vi "CAPCartTopLevelV2.vi"() -> ()   [LabVIEW 2020]
uses:
  <vilib>/Utility/file.llb/Read Delimited Spreadsheet (string).vi
  BK Precision 4050B Series/BK Precision 4050B Series.lvlib
  consol_upload3 2020/consol_upload3 2020/Program Files/National Instruments/LabVIEW 2021/instr.lib/BK Precision 9200 Series/BK Precision 9200 Series.lvlib
  CAPCart LabVIEW/Marlin/Marlin.lvlib
  Ocean Optics 2000 4000/Ocean Optics 2000 4000.lvlib
panel:
  in  "Flow Controller":refnum<visa-resource-name>="Alicat"
  in  "Enable Strobe (Disabled)":bool
  out "Spectral Waveform":cluster{dbl[], dbl[]}(graph)
  in  "Stop":bool
  in  "Spectrometer":refnum<visa-resource-name>
  out "Frequency Command":string
  out "Voltage Command":string
  out "XYZ Command":string
  out "Flow Command":string
  in  "Time per measurement (ms)":u32
  in  "?":bool
  in  "File path (dialog if empty)":path
  in  "3D Printer":refnum<visa-resource-name>
  in  "Voltage Limit (66V)":dbl=66.0 format="%.2f"
  in  "Enable OVP (T: Enable) 2":bool=TRUE
  in  "Current Limit (1.0 A)":dbl=1.0 format="%.3g"
  in  "Power Supply":refnum<visa-resource-name>
  in  "Function Generator 2":refnum<visa-resource-name>="COM9"
  in  "Amplitude  2":dbl=1.0 format="%#.3f"
  in  "DC Offset (0.00 V)":dbl
  in  "Pulse Width/Duty (20%)":dbl=20.0 format="%.3g"
  # "Plasma and Electric Space Propulsion Lab\nOregon State University\nAlexander Reed & Blake Haist\n\nCAPCartTopLevelRev5.14"
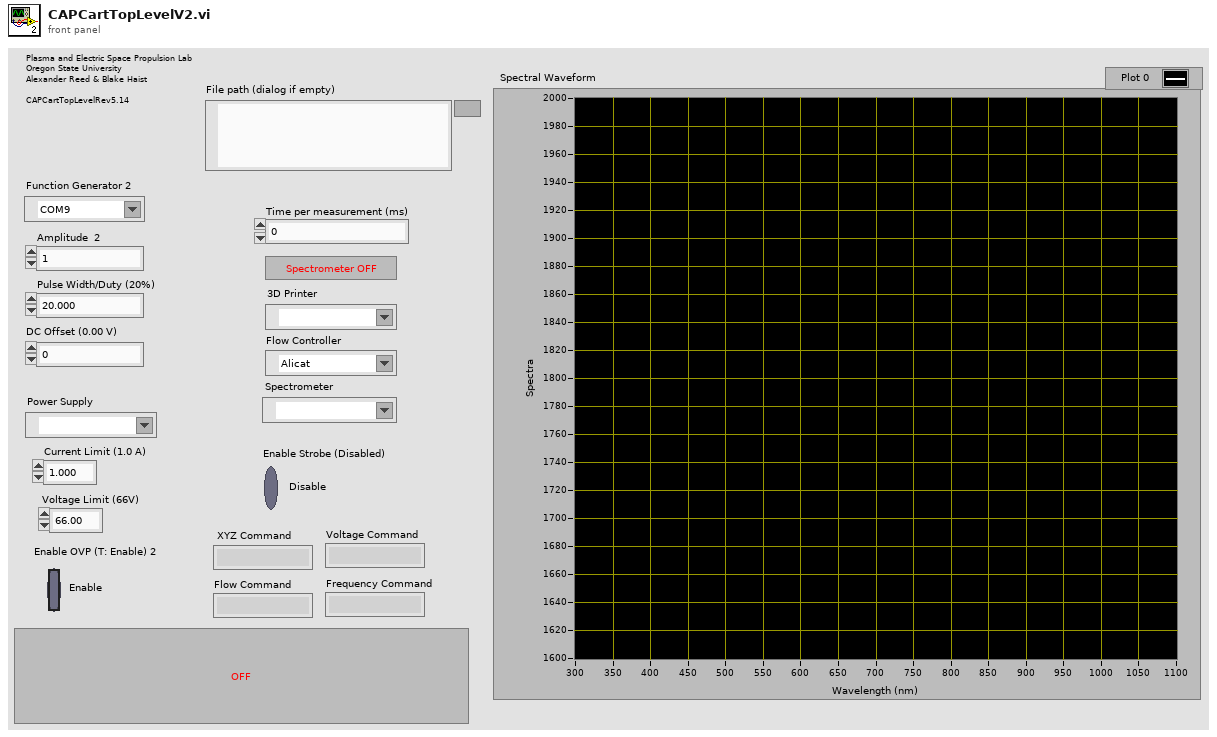
[diagram p1: front panel]
types:
  T1 = cluster{"Wavelength (nm)":dbl[], "Spectrum by Pixel Number":dbl[]}
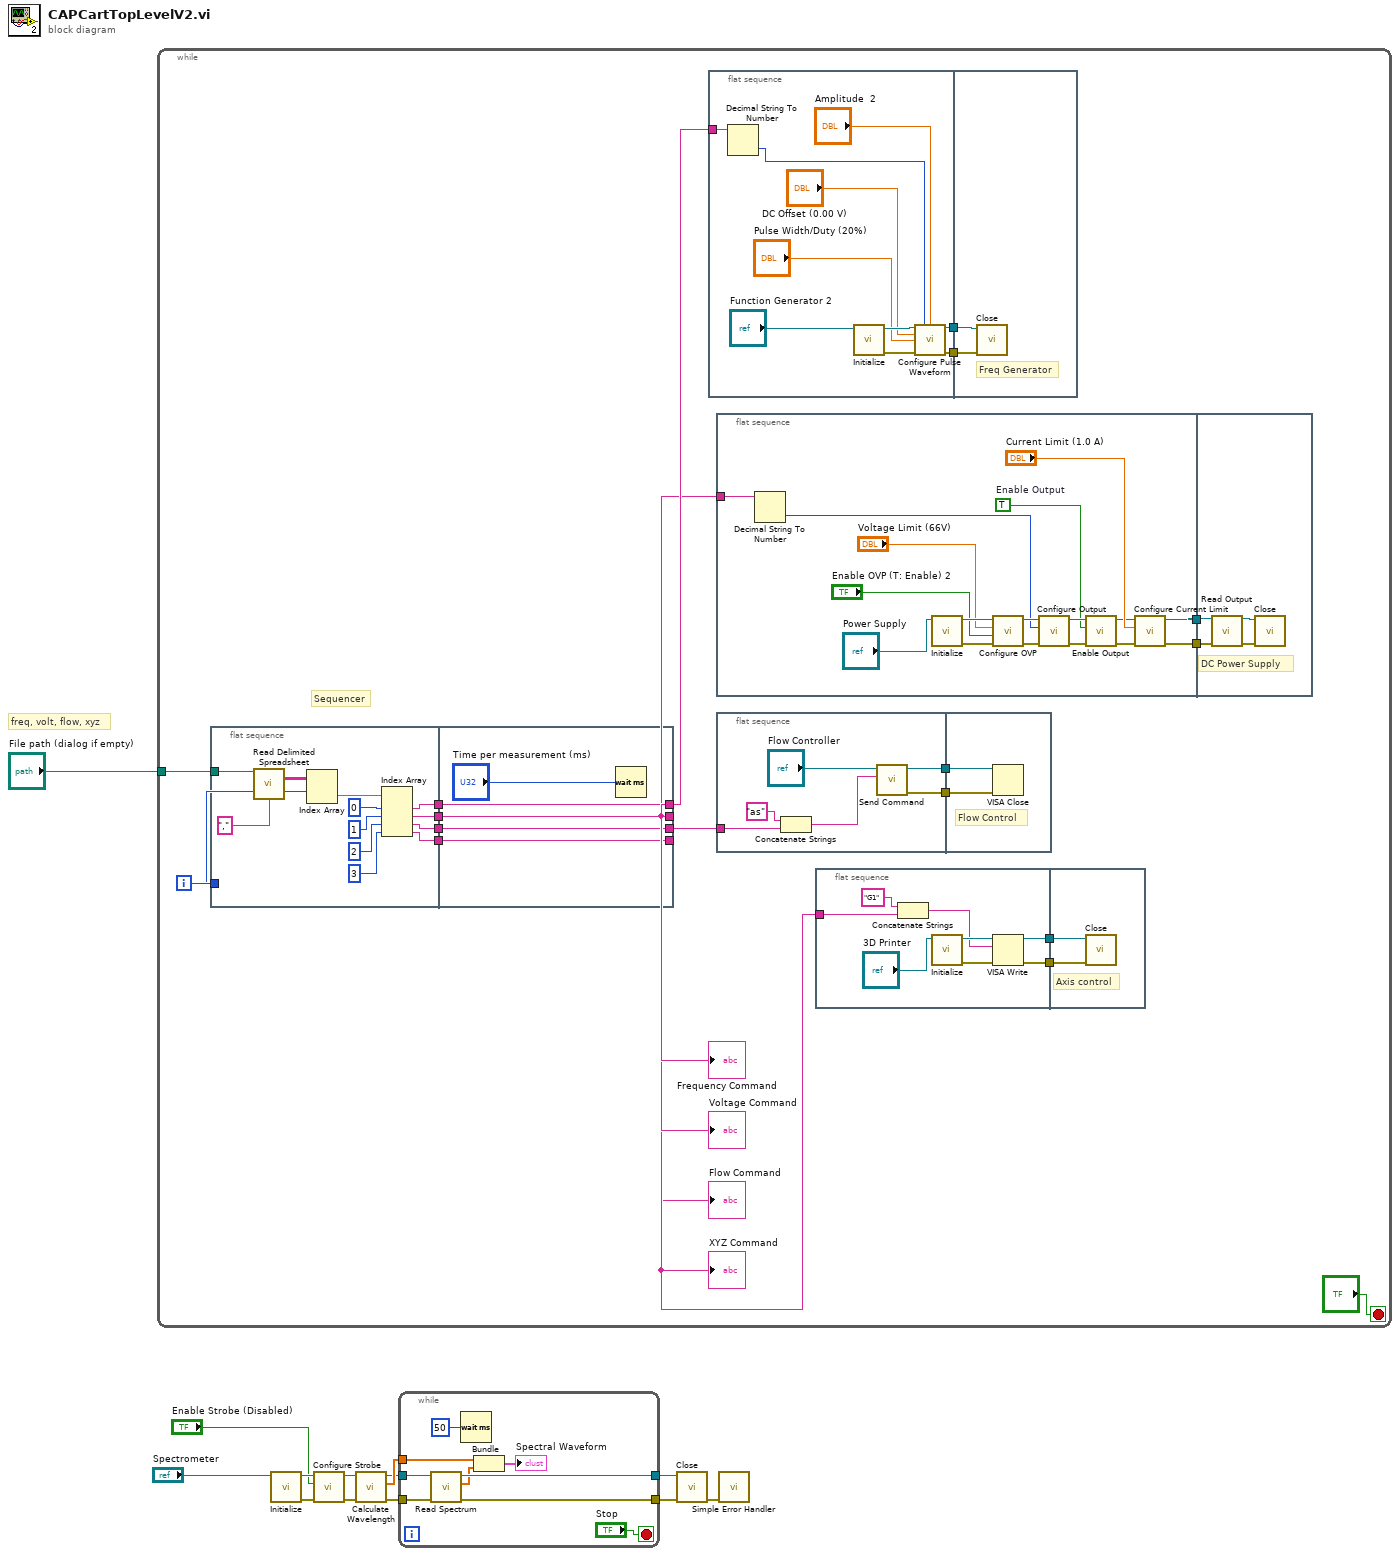
[diagram p0: block diagram]
diagram:
  # "freq, volt, flow, xyz"
  n1 = while {
    tunnel: "File path (dialog if empty)" -> [w28]
    i -> [w27]
    stop <- "?" stop-if-true
    # "Sequencer"
    n2 = flat-sequence {
      tunnel: w28 -> [w96]
      tunnel: [w88] -> w32
      tunnel: [w87] -> w31
      tunnel: [w86] -> w30
      tunnel: [w85] -> w29
      tunnel: w27 -> [w93]
      tunnel: w32 -> [w100]
      tunnel: [w100] -> w19
      tunnel: w31 -> [w99]
      tunnel: [w99] -> w18
      tunnel: w30 -> [w97]
      tunnel: w29 -> [w98]
      tunnel: [w98] -> w17
      tunnel: [w97] -> w16
      frame #0 {
        n3 = call-poly <vilib>:"Read Delimited Spreadsheet.vi"("file path (dialog if empty)"=w96, "delimiter (\\t)"="," ("delimiter (\\t)")) -> ("all rows"=w95:string[][])  [unwired: 8 in, 5 out]
        n4 = Index Array(array=w95, index (row)=w93) -> (element=w94:string[])  [unwired: 1 in]
        n5 = Index Array(array=w94, index #1=0 ("index"), index #2=1 ("index"), index #3=2 ("index"), index #4=3 ("index")) -> (element #1=w88:string, element #2=w87:string, element #3=w86:string, element #4=w85:string)
      }
      frame #1 {
        n6 = Wait (ms)(milliseconds to wait="Time per measurement (ms)") -> ()  [unwired: 1 out]
      }
    }
    n7 = flat-sequence {
      tunnel: [w75] -> w25
      tunnel: [w74] -> w24
      tunnel: w19 -> [w73]
      tunnel: w25 -> [w83]
      tunnel: w24 -> [w82]
      frame #0 {
        n8 = Decimal String To Number(string=w73) -> (number=w72:i32)  [unwired: 2 in, 1 out]
        n9 = call "Initialize.vi"("VISA resource name"="Function Generator 2") -> ("error out"=w79:errorcluster, "VISA resource name out"=w80:refnum<visa-resource-name>)  [unwired: 9 in]
        n10 = call "Configure Pulse Waveform.vi"("VISA resource name"=w80, "Frequency (1000 Hz)"=w72, "Amplitude (1.0 Vpp)"="Amplitude  2", "DC Offset (0.00 V)"="DC Offset (0.00 V)", "Pulse Width/Duty (20%)"="Pulse Width/Duty (20%)", "error in (no error)"=w79) -> ("VISA resource name out"=w75:refnum<visa-resource-name>, "error out"=w74:errorcluster)  [unwired: 8 in]
      }
      frame #1 {
        # "Freq Generator"
        n11 = call "Close.vi"("error in (no error)"=w82, "VISA resource name"=w83) -> ()  [unwired: 9 in, 1 out]
      }
    }
    n12 = flat-sequence {
      tunnel: [w54] -> w23
      tunnel: [w53] -> w22
      tunnel: w18 -> [w52]
      tunnel: w23 -> [w71]
      tunnel: w22 -> [w70]
      frame #0 {
        w56 = TRUE  # Enable Output
        n13 = Decimal String To Number(string=w52) -> (number=w51:i32)  [unwired: 2 in, 1 out]
        n14 = call "Initialize.vi"("VISA resource name"="Power Supply") -> ("error out"=w67:errorcluster, "VISA resource name out"=w66:refnum<visa-resource-name>)  [unwired: 9 in]
        n15 = call "Configure OVP.vi"("error in (no error)"=w67, "Enable OVP (T: Enable)"="Enable OVP (T: Enable) 2", "Voltage Limit (66.000 V)"="Voltage Limit (66V)", "VISA resource name"=w66) -> ("error out"=w63:errorcluster, "VISA resource name out"=w64:refnum<visa-resource-name>)  [unwired: 6 in]
        n16 = call "Configure Output.vi"("error in (no error)"=w63, "Voltage Level (0.0 V)"=w51, "VISA resource name"=w64) -> ("error out"=w59:errorcluster, "VISA resource name out"=w60:refnum<visa-resource-name>)  [unwired: 7 in]
        n17 = call "Enable Output.vi"("error in (no error)"=w59, "Enable Output (F: False)"=w56, "VISA resource name"=w60) -> ("error out"=w58:errorcluster, "VISA resource name out"=w57:refnum<visa-resource-name>)  [unwired: 7 in]
        n18 = call "Configure Current Limit.vi"("error in (no error)"=w58, "Current Limit (0.0 A)"="Current Limit (1.0 A)", "VISA resource name"=w57) -> ("error out"=w53:errorcluster, "VISA resource name out"=w54:refnum<visa-resource-name>)  [unwired: 7 in]
      }
      frame #1 {
        # "DC Power Supply"
        n19 = call "Read Output.vi"("VISA resource name"=w71, "error in (no error)"=w70) -> ("VISA resource name out"=w69:refnum<visa-resource-name>, "error out"=w68:errorcluster)  [unwired: 9 in, 3 out]
        n20 = call "Close.vi"("error in (no error)"=w68, "VISA resource name"=w69) -> ()  [unwired: 9 in, 1 out]
      }
    }
    n21 = flat-sequence {
      tunnel: w16 -> [w36]
      tunnel: [w37] -> w15
      tunnel: [w38] -> w14
      tunnel: w15 -> [w40]
      tunnel: w14 -> [w39]
      frame #0 {
        n22 = Concatenate Strings("as" ("string"), w36) -> (w35:string)
        n23 = call "Send Command.vi"("Command"=w35, "VISA Session In"="Flow Controller") -> ("error out"=w38:errorcluster, "VISA Session Out"=w37:refnum<visa-resource-name>)  [unwired: 7 in, 1 out]
      }
      frame #1 {
        # "Flow Control"
        n24 = VISA Close(VISA resource name=w40, error in (no error)=w39) -> ()  [unwired: 1 out]
      }
    }
    n25 = flat-sequence {
      tunnel: [w44] -> w21
      tunnel: [w46] -> w20
      tunnel: w17 -> [w42]
      tunnel: w21 -> [w49]
      tunnel: w20 -> [w50]
      frame #0 {
        n26 = Concatenate Strings("G1" ("string"), w42) -> (w41:string)
        n27 = call "Initialize.vi"("VISA resource name"="3D Printer") -> ("error out"=w45:errorcluster, "VISA resource name out"=w47:refnum<visa-resource-name>)  [unwired: 9 in]
        n28 = VISA Write(VISA resource name=w47, write buffer=w41, error in (no error)=w45) -> (VISA resource name out=w46:refnum<visa-resource-name>, error out=w44:errorcluster)  [unwired: 1 out]
      }
      frame #1 {
        # "Axis control"
        n29 = call "Close.vi"("error in (no error)"=w49, "VISA resource name"=w50) -> ()  [unwired: 9 in, 1 out]
      }
    }
    "Flow Command" <- w16
    "XYZ Command" <- w17
    "Voltage Command" <- w18
    "Frequency Command" <- w19
  }
  n30 = call "Initialize.vi"("VISA resource name"="Spectrometer") -> ("error out"=w11:errorcluster, "VISA resource name out"=w12:refnum<visa-resource-name>)  [unwired: 2 in, 7 out]
  n31 = call "Configure Strobe.vi"("error in (no error)"=w11, "Enable Strobe (Disabled)"="Enable Strobe (Disabled)", "VISA resource name"=w12) -> ("error out"=w1:errorcluster, "VISA resource name out"=w2:refnum<visa-resource-name>)  [unwired: 7 out]
  n32 = call "Calculate Wavelength.vi"("error in (no error)"=w1, "VISA resource name"=w2) -> ("error out"=w3:errorcluster, "Wavelength (nm)"=w5:dbl[], "VISA resource name out"=w4:refnum<visa-resource-name>)  [unwired: 1 in, 6 out]
  n33 = while {
    tunnel: [w108] -> w9
    tunnel: [w107] -> w8
    tunnel: w5 -> [w106]
    tunnel: w4 -> [w104]
    tunnel: w3 -> [w103]
    stop <- "Stop" stop-if-true
    n34 = call "Read Spectrum.vi"("error in (no error)"=w103, "VISA resource name"=w104) -> ("error out"=w107:errorcluster, "Spectrum by Pixel Number"=w105:dbl[], "VISA resource name out"=w108:refnum<visa-resource-name>)  [unwired: 6 in, 1 out]
    n35 = Wait (ms)(milliseconds to wait=u32 50 ("millisecond multiple")) -> ()  [unwired: 1 out]
    n36 = Bundle("Wavelength (nm)"=w106, "Spectrum by Pixel Number"=w105) -> (→"Spectral Waveform":T1)  [unwired: 1 out]
  }
  n37 = call "Close.vi"("error in (no error)"=w8, "VISA resource name"=w9) -> ("error out"=w7:errorcluster)  [unwired: 9 out]
  n38 = call <vilib>:"Simple Error Handler.vi"("error in (no error)"=w7) -> ()  [unwired: 1 in, 8 out]
